vi "ADC SNR_original.vi"(8 "error in (no error)":errorcluster, 9 "Sequence parameters":string[][](array[string])=[["Min limit", "Max limit", "Register sheet file", "Register Sheet"], ["", "", "CC2600.xls", "TX_BLE;Trim"], ["Reg write (addr;value)", "Operating frequency [Hz]", "", ""], ["NA", "2.44G", "", ""]], 10 "Run type":i32, 11 "Method parameters":T4={"Dev"={"Do not disturb DUT"=FALSE, "XOSC"=32000000.0, "Board type"="", "EM"="", "Configure tempboard"=TRUE, "Device specific info"=[], "Generic Object"=refnum}, "Method"={"Run type"=1, "Test name"="Current LPM2 4", "Comment"="", "Results folder"="", "AFC"=enum."Off", "Method name"="Current LPM2 4", "Method results"={"Excel brief report"=FALSE, "Spotfire report"=FALSE, "Starfish report"=FALSE}, "Operator"="", "Reference time"=timestamp(0 s since 1904-01-01), "AFC delay"=0.0, "Initialization"=enum."Enabled", "MD5 Sum"="", "HW addon board"=enum."None", "AFC Regsheet"="", "AFC Regfile"=path "", "dummy"=0.0}, "Inst"={"Instr"={"PS1"={"Name"="", "GPIB address"="", "VISA session"=""}, "PS2"={"Name"="", "GPIB address"="", "VISA session"=""}, "TC1"={"Name"="", "GPIB address"="", "VISA session"=""}, "TC2"={"Name"="", "GPIB address"="", "VISA session"=""}, "SA1"={"Name"="", "GPIB address"="", "VISA session"=""}, "SA2"={"Name"="", "GPIB address"="", "VISA session"=""}, "SG1"={"Name"="", "GPIB address"="", "VISA session"=""}, "SG2"={"Name"="", "GPIB address"="", "VISA session"=""}, "SG3"={"Name"="", "GPIB address"="", "VISA session"=""}, "MI1"={"Name"="", "GPIB address"="", "VISA session"=""}, "MI2"={"Name"="", "GPIB address"="", "VISA session"=""}, "SW SA"={"Name"="", "Controller addr"=""}, "SW SG"={"Name"="", "Controller addr"=""}, "MI3"={"Name"="", "GPIB address"="", "VISA session"=""}}, "Switchbox"={"RF Path"=0, "Cal compensation"=enum."TX", "Switchbox gain mode"="", "State"=enum."TX"}, "Instr to control (i.e. SA1)"="Default", "Intrument info string"=""}, "Sequence parameters"=[["Weight", "Min Limit", "Max Limit", "Register Sheet", "", "", "", "", "", "", "", "", ""], ["Vital", "", "1", "LPM2", "", "", "", "", "", "", "", "", ""], ["Resolution", "Reg write (addr;value)", "Chip mode", "Range", "", "", "", "", "", "", "", "", ""], ["u", "NA", "", "auto", "", "", "", "", "", "", "", "", ""]], "Cond"={"Temp logged"=25.0, "VDD1_PS1_6V"=-999.0, "VDD2_PS1_25V"=-999.0, "VDD4_PS2_25V"=-999.0, "VDD3_PS2_6V"=-999.0}, "Meas config"={"X-axis inner loop index"=32000000, "Y-axis outer loop index"=32000000, "X-axis"=[], "Y-axis"=[], "X-axis array req size"=32000000, "Y-axis array req size"=32000000, "Param description"=[], "Use meas clust for reporting"=FALSE, "Parameter index (page)"=0, "X-axis name"="", "Y-axis name"=""}} {"Cond"."VDD3_PS2_6V" format="%.3f"; "Cond"."VDD4_PS2_25V" format="%.3f"; "Cond"."VDD2_PS1_25V" format="%.3f"; "Cond"."VDD1_PS1_6V" format="%.3f"; "Method"."dummy" format="%.1p"; "Method"."AFC delay" format="%.1p"; "Dev"."XOSC" format="%.3p"}) -> (0 "error out":errorcluster, 1 "End method error":T3, 3 "Result summary":string[][](array[string])=[["Critical", "Output Power@2405 MHz", "-3", "4", "dBm"], ["Critical", "Output Power@2410 MHz", "-3", "4", "dBm"]])   [LabVIEW 2019]
doc: "[AutoDocStart]Performs crystal accuracy measurements. Measures the offset from ideal frequency. Primarily used for tuning XOSC capacitors and verifying XOSC trims.\n\nSweeping parameters: operating frequency, OSC override value and VDDR level\n\nResults: Offset frequency in ppm[AutoDocEnd]"
uses:
  User Lib/Utilities/Cluster definitions/DUT VDD1.ctl
  User Lib/Utilities/Cluster definitions/DUT VDD2.ctl
  User Lib/Utilities/Cluster definitions/DUT VDD3.ctl
  User Lib/Utilities/Cluster definitions/DUT VDD4.ctl
  User Lib/Utilities/Cluster definitions/DUT vdd control.ctl
  User Lib/Utilities/Cluster definitions/Instr clust.ctl
  User Lib/Utilities/Cluster definitions/Method input.ctl
  User Lib/Utilities/Controls/Automatic Frequency Compensation types.ctl
  User Lib/Utilities/Controls/Method Reports.ctl
  User Lib/Utilities/Cluster definitions/End method error cluster.ctl
  User Lib/Utilities/Cluster definitions/Device specific info.ctl
  User Lib/Utilities/Cluster definitions/Method Initialization.ctl
  User Lib/Utilities/Switchbox control/SwitchBox_State._ENUMctl.ctl
  User Lib/Utilities/Controls/HW addon boards.ctl
panel:
  in  "path to save":T1={"Path to Save plot"=path "D:/Tenor_176P/DYN_PAR_C004/DAT/D001_TEMPP30C_VDD1.2_VDDA3.3_16B_SE_ADCA__vicA_aggX_PLT_CAP_200821_1740_33.jpg", "Path to Raw Data plot"=path "D:/Tenor_176P/DYN_PAR_C004/DAT/D001_TEMPP30C_VDD1.2_VDDA3.3_16B_SE_ADCA__vicA_aggX_RAW_DAT_200821_1740_33.csv"}
  in  "Tab Control":T2(tab)
  out "Dynamic Parameters":T12={"SNR"=nan, "SNRD"=nan, "THD"=nan, "ENOB (SNRD)"=nan, "SFDR"=nan, "ENOB (SNR)"=nan, "Noise Power"=nan, "Signal power"=nan} {"Signal power" format="%.6f"; "Noise Power" format="%.2f"; "ENOB (SNR)" format="%.2f"; "SFDR" format="%.2f"; "ENOB (SNRD)" format="%.2f"; "THD" format="%.2f"; "SNRD" format="%.2f"; "SNR" format="%.2f"}
  # "°C"
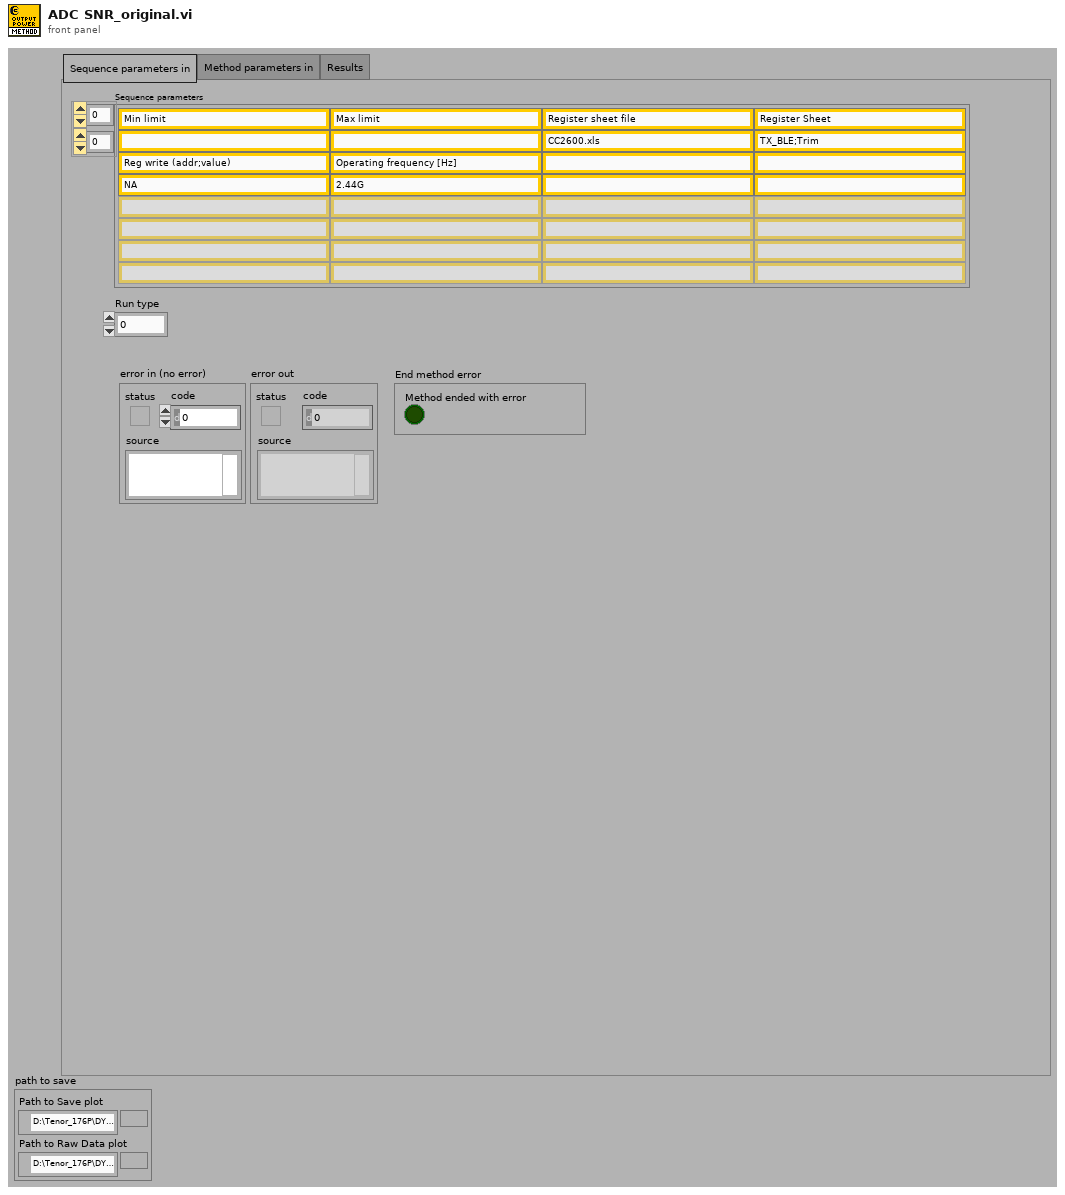
[diagram p1: front panel]
types:
  T1 = cluster{"Path to Save plot":path, "Path to Raw Data plot":path}
  T2 = enum32{"Sequence parameters in", "Method parameters in", "Results"}
  T3 = typedef "End method error cluster.ctl" = cluster{"Method ended with error":bool}
  T4 = typedef "Method input.ctl" = cluster{"Dev":cluster{"Do not disturb DUT":bool, "XOSC":dbl, "Board type":string, "EM":string, "Configure tempboard":bool, "Device specific info":T5[], "Generic Object":refnum<class>}, "Method":cluster{"Run type":i32, "Test name":string, "Comment":string, "Results folder":string, "AFC":T6, "Method name":string, "Method results":T7, "Operator":string, "Reference time":timestamp, "AFC delay":dbl, "Initialization":T8, "MD5 Sum":string, "HW addon board":T9, "AFC Regsheet":string, "AFC Regfile":path, "dummy":dbl}, "Inst":T10, "Sequence parameters":string[][], "Cond":cluster{"Temp logged":dbl, "VDD1_PS1_6V":dbl, "VDD2_PS1_25V":dbl, "VDD4_PS2_25V":dbl, "VDD3_PS2_6V":dbl}, "Meas config":cluster{"X-axis inner loop index":i32, "Y-axis outer loop index":i32, "X-axis":string[], "Y-axis":string[], "X-axis array req size":i32, "Y-axis array req size":i32, "Param description":string[][], "Use meas clust for reporting":bool, "Parameter index (page)":i32, "X-axis name":string, "Y-axis name":string}}
  T5 = typedef "Device specific info.ctl" = cluster{"EM number":u8, "IP address":string, "Enabled":bool, "Slot no":u8, "RF path":u8, "EM name":string, "Wafer info":string, "AFC frequency ppm":dbl, "Register writes":string[][], "Meas data":string[][][], "Device comment":string}
  T6 = typedef "Automatic Frequency Compensation types.ctl" = enum16{"Off", "Compensate Instrument frequency", "Compensate DUT frequency", "Predictive - Compensate Instrument frequency", "Predictive - Compensate DUT frequency", "Do not skip re-init - Compensate Instrument frequency", "Do not skip re-init - Compensate DUT frequency"}
  T7 = typedef "Method Reports.ctl" = cluster{"Excel brief report":bool, "Spotfire report":bool, "Starfish report":bool}
  T8 = typedef "Method Initialization.ctl" = enum16{"Enabled", "Skip Instr and Device Init", "Enabled with Separate Flash", "Set PS, Device Init and Skip Instr Init", "Skip Device Init"}
  T9 = typedef "HW addon boards.ctl" = enum16{"None", "Current meas 5EM", "Stresstest 10EM"}
  T10 = typedef "Instr clust.ctl" = cluster{"Instr":cluster{"PS1":cluster{"Name":string, "GPIB address":string, "VISA session":refnum<visa-resource-name>}, "PS2":cluster{"Name":string, "GPIB address":string, "VISA session":refnum<visa-resource-name>}, "TC1":cluster{"Name":string, "GPIB address":string, "VISA session":refnum<visa-resource-name>}, "TC2":cluster{"Name":string, "GPIB address":string, "VISA session":refnum<visa-resource-name>}, "SA1":cluster{"Name":string, "GPIB address":string, "VISA session":refnum<visa-resource-name>}, "SA2":cluster{"Name":string, "GPIB address":string, "VISA session":refnum<visa-resource-name>}, "SG1":cluster{"Name":string, "GPIB address":string, "VISA session":refnum<visa-resource-name>}, "SG2":cluster{"Name":string, "GPIB address":string, "VISA session":refnum<visa-resource-name>}, "SG3":cluster{"Name":string, "GPIB address":string, "VISA session":refnum<visa-resource-name>}, "MI1":cluster{"Name":string, "GPIB address":string, "VISA session":refnum<visa-resource-name>}, "MI2":cluster{"Name":string, "GPIB address":string, "VISA session":refnum<visa-resource-name>}, "SW SA":cluster{"Name":string, "Controller addr":string}, "SW SG":cluster{"Name":string, "Controller addr":string}, "MI3":cluster{"Name":string, "GPIB address":string, "VISA session":refnum<visa-resource-name>}}, "Switchbox":cluster{"RF Path":i32, "Cal compensation":enum16{"TX", "RX", "Interferer", "No compensation", "Interferer2"}, "Switchbox gain mode":string, "State":T11}, "Instr to control (i.e. SA1)":string, "Intrument info string":string}
  T11 = typedef "SwitchBox_State._ENUMctl.ctl" = enum16{"TX", "RX", "SP:TX", "SP:RX", "SW:TX", "SW:RX"}
  T12 = cluster{"SNR":dbl, "SNRD":dbl, "THD":dbl, "ENOB (SNRD)":dbl, "SFDR":dbl, "ENOB (SNR)":dbl, "Noise Power":dbl, "Signal power":dbl}
  T13 = cluster{"Save INL/DNL Plot(Ramp)":bool, "Save SNR Plot":bool, "Save INL/DNL Plot(Sine)":bool, "Save INL/DNL Raw Data(Ramp)":bool, "Save SNR Raw Data":bool, "Save INL/DNL Raw Data(Sine)":bool, "Save DC Raw data":bool, "Save  Raw Data(Sine)":bool}
  T14 = cluster{"Fundamental Frequency":dbl, "Sampling Frequncy":dbl, "No of Harmonics":u8, "Window":enum16{"None ", "Hanning", "Hamming", "Blackman-Harris", "Exact Blackman", "Blackman", "Flat Top", "4 Term B-Harris ", "7 Term B-Harris"}, "Blackman (fundamental power) bins)":dbl}
  T15 = typedef "DUT vdd control.ctl" = cluster{"VDD4 config":T16, "VDD3 config":T17, "VDD2 config":T18, "VDD1 config":T19}
  T16 = typedef "DUT VDD4.ctl" = u16
  T17 = typedef "DUT VDD3.ctl" = u16
  T18 = typedef "DUT VDD2.ctl" = u16
  T19 = typedef "DUT VDD1.ctl" = u16
  T20 = enum32{"NI Card Settings", "Memory Read Setting", "DC Capture", "ADC Ramp", "ADC Sine", "SNR", "Cap Calibration"}
  T21 = enum32{"Read from Memory", "Read .dat file", "NI Card Capture", "None"}
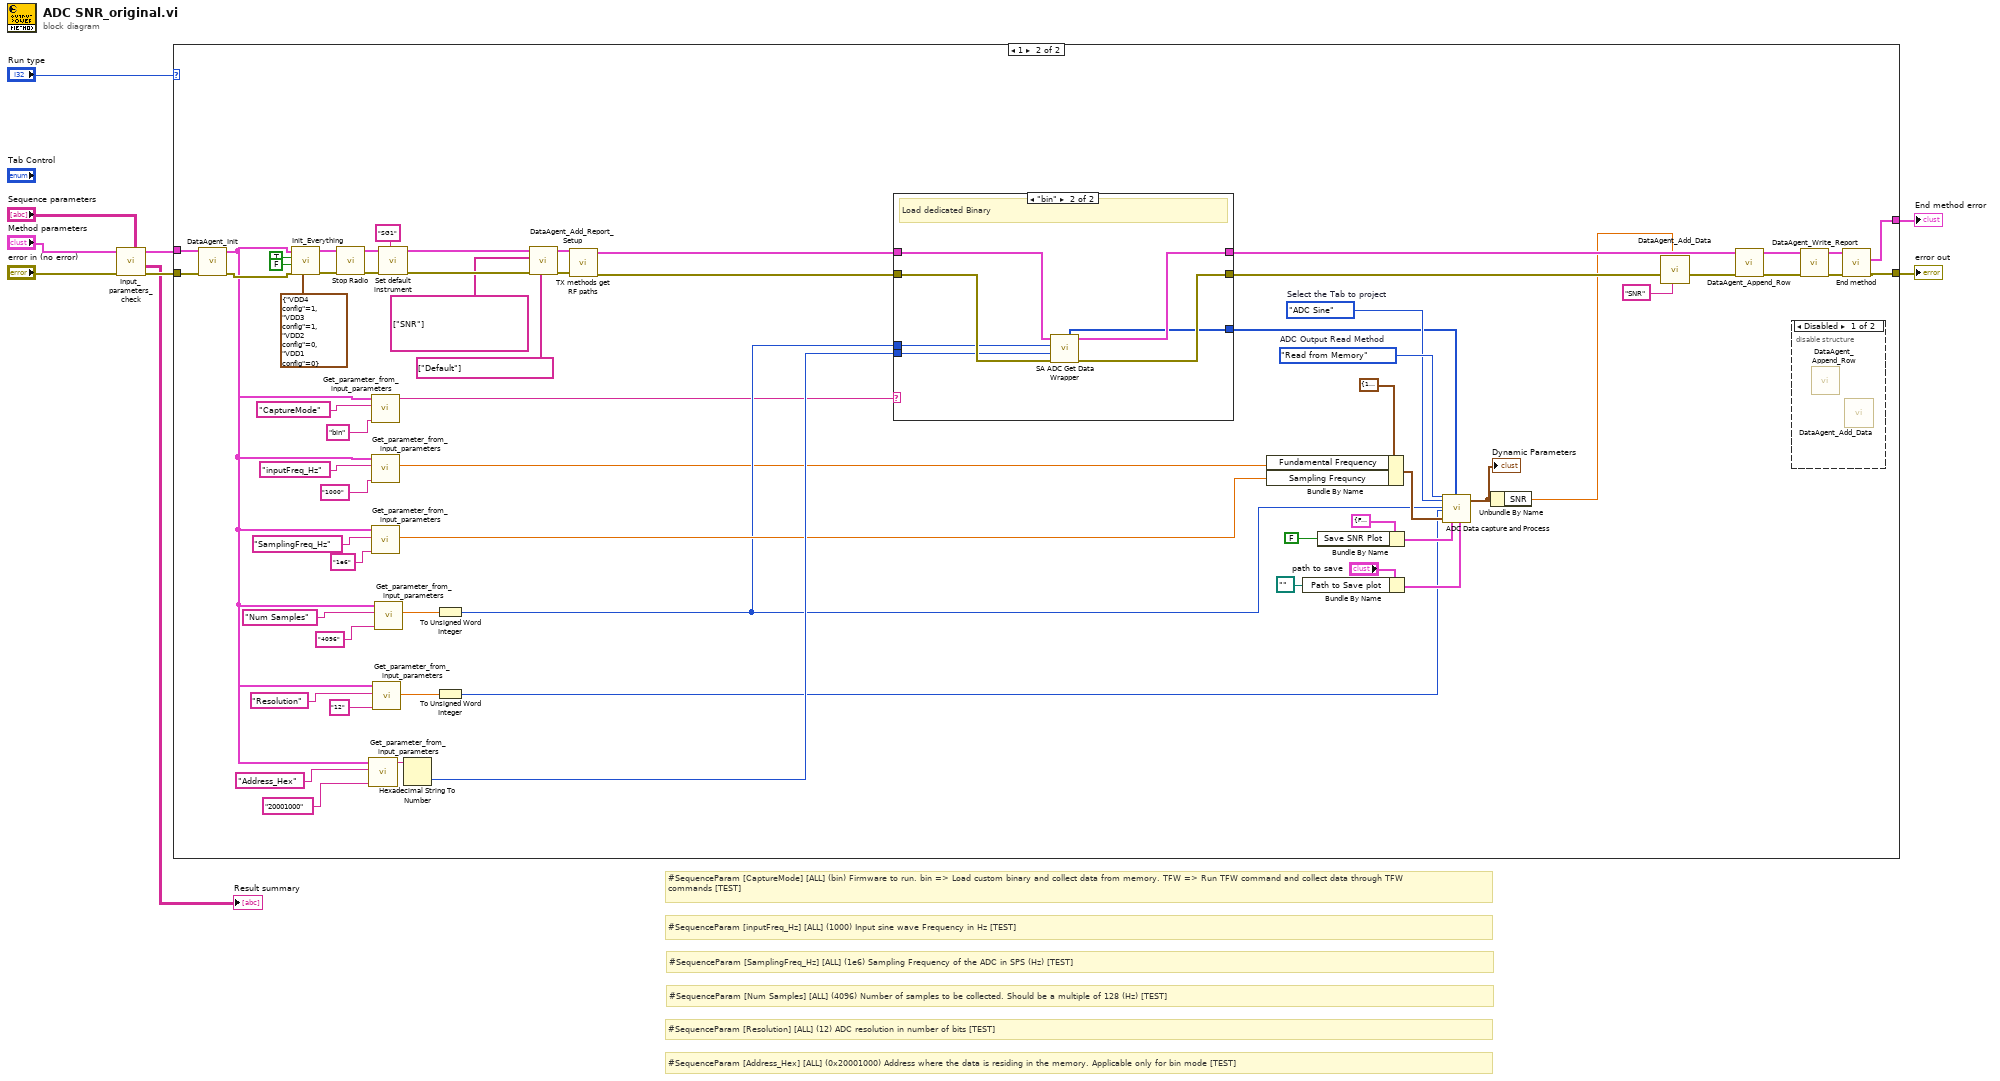
[diagram p0: block diagram]
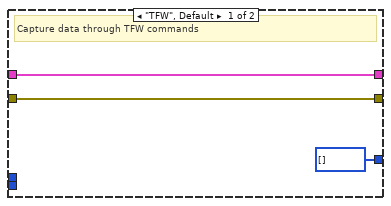
[diagram p3: hidden frame]
diagram:
  # "#SequenceParam [CaptureMode] [ALL] (bin) Firmware to run. bin => Load custom binary and collect data from memory. TFW => Run TFW command and collect data through TFW commands [TEST]"
  # "#SequenceParam [Address_Hex] [ALL] (0x20001000) Address where the data is residing in the memory. Applicable only for bin mode [TEST]"
  # "#SequenceParam [Resolution] [ALL] (12) ADC resolution in number of bits [TEST]"
  # "#SequenceParam [Num Samples] [ALL] (4096) Number of samples to be collected. Should be a multiple of 128 (Hz) [TEST]"
  # "#SequenceParam [SamplingFreq_Hz] [ALL] (1e6) Sampling Frequency of the ADC in SPS (Hz) [TEST]"
  # "#SequenceParam [inputFreq_Hz] [ALL] (1000) Input sine wave Frequency in Hz [TEST]"
  n1 = call "Input_parameters_check.vi"("Sequence parameters"="Sequence parameters", "error in"="error in (no error)", "Method cluster in"="Method parameters") -> ("error out"=w8:errorcluster, "Result summary"=→"Result summary":string[][], "Method cluster out"=w4:T4)  [unwired: 6 in]
  n2 = case shown="1" "Run type" {
    tunnel: w8 -> [w10 w67]
    tunnel: [w10 w74] -> w9
    tunnel: w4 -> [_ w68]
    tunnel: [_ w73] -> w3
    frame 0, Default {
      # "Run type 0 is only for formatting the result summary"
    }
    frame 1 {
      w37 = T20."ADC Sine"  # Select the Tab to project
      w38 = T21."Read from Memory"  # ADC Output Read Method
      n3 = call "DataAgent_Init.vi"("error in (no error)"=w67, "Method cluster in"=w68) -> ("error out"=w66:errorcluster, "Method cluster out"=w20:T4)  [unwired: 8 in]
      n4 = call "Init_Everything.vi"("VDD config"=T15 {"VDD4 config"=1, "VDD3 config"=1, "VDD2 config"=0, "VDD1 config"=0}, "error in"=w66, "Support current measurement?"=FALSE, "Override VDD Config"=TRUE, "Method cluster In"=w20) -> ("error out"=w59:errorcluster, "Method cluster out"=w56:T4)  [unwired: 3 in, 2 out]
      n5 = call "Stop Radio.vi"("error in (no error)"=w59, "Method cluster in"=w56) -> ("error out"=w58:errorcluster, "Method cluster out"=w57:T4)  [unwired: 8 in]
      n6 = call "Get_parameter_from_input_parameters.vi"("Default value (used if not specified on Front Panel)"="20001000", "Parameter name"="Address_Hex" ("SA_ param name"), "Method cluster (if input param empty)"=w20) -> ("value as String"=w43:string)  [unwired: 2 in, 6 out]
      n7 = call "Get_parameter_from_input_parameters.vi"("Default value (used if not specified on Front Panel)"="bin", "Parameter name"="CaptureMode" ("SA_ param name"), "Method cluster (if input param empty)"=w20) -> ("value as String"=w19:string)  [unwired: 2 in, 6 out]
      n8 = call "Get_parameter_from_input_parameters.vi"("Default value (used if not specified on Front Panel)"="1000", "Parameter name"="inputFreq_Hz" ("SA_ param name"), "Method cluster (if input param empty)"=w20) -> ("value as DBL"=w23:dbl)  [unwired: 2 in, 6 out]
      n9 = call "Get_parameter_from_input_parameters.vi"("Default value (used if not specified on Front Panel)"="1e6", "Parameter name"="SamplingFreq_Hz" ("SA_ param name"), "Method cluster (if input param empty)"=w20) -> ("value as DBL"=w39:dbl)  [unwired: 2 in, 6 out]
      n10 = call "Get_parameter_from_input_parameters.vi"("Default value (used if not specified on Front Panel)"="12", "Parameter name"="Resolution" ("SA_ param name"), "Method cluster (if input param empty)"=w20) -> ("value as DBL"=w45:dbl)  [unwired: 2 in, 6 out]
      n11 = call "Get_parameter_from_input_parameters.vi"("Default value (used if not specified on Front Panel)"="4096", "Parameter name"="Num Samples" ("SA_ param name"), "Method cluster (if input param empty)"=w20) -> ("value as DBL"=w44:dbl)  [unwired: 2 in, 6 out]
      n12 = call "Set default instrument.vi"("Default value (used if not specified on Front Panel)"="SG1", "error in (no error)"=w58, "Method cluster in"=w57) -> ("error out"=w65:errorcluster, "Method cluster out"=w64:T4)  [unwired: 7 in]
      n13 = Hexadecimal String To Number(string=w43) -> (number=w42:u32)  [unwired: 2 in, 1 out]
      n14 = To Unsigned Word Integer(number=w44) -> (unsigned 16bit integer=w27:u16)
      n15 = To Unsigned Word Integer(number=w45) -> (unsigned 16bit integer=w26:u16)
      n16 = call "DataAgent_Add_Report_Setup.vi"("Y-axis Titles"=string[] ["Default"], "error in (no error)"=w65, "Loop parameter names"=string[] ["SNR"], "Method cluster in"=w64) -> ("error out"=w52:errorcluster, "Method cluster out"=w53:T4)  [unwired: 3 in, 3 out]
      n17 = call "TX methods get RF paths.vi"("error in (no error)"=w52, "Method clust in"=w53) -> ("error out"=w55:errorcluster, "Method clust out"=w54:T4)  [unwired: 7 in, 1 out]
      n18 = case shown="\"bin\"" w19 {
        tunnel: [w77 w84] -> w18
        tunnel: [w76 w83] -> w15
        tunnel: w55 -> [w76 w82]
        tunnel: w54 -> [w77 w81]
        tunnel: w42 -> [_ w80]
        tunnel: [u32[] [] ("ADC samples") w79] -> w31
        tunnel: w27 -> [_ w78]
        frame "TFW", Default {
          # "Capture data through TFW commands"
        }
        frame "bin" {
          # "Load dedicated Binary"
          n19 = call "SA ADC Get Data Wrapper.vi"("error in"=w82, "Data Address"=w80, "Num Samples"=w78, "Method cluster in"=w81) -> ("error out"=w83:errorcluster, "output cluster"=w84:T4, "ADC samples"=w79:u32[])  [unwired: 2 in, 3 out]
        }
      }
      n20 = Bundle By Name(cluster=T14 {"Fundamental Frequency"=100000.0, "Sampling Frequncy"=3999610.0, "No of Harmonics"=9, "Window"=enum."7 Term B-Harris", "Blackman (fundamental power) bins)"=1.0} ("Inputs for Dyanmic para"), "Fundamental Frequency"=w23, "Sampling Frequncy"=w39) -> (w34:T14)
      n21 = Bundle By Name(cluster="path to save", "Path to Save plot"=path "") -> (w29:T1)
      n22 = Bundle By Name(cluster=T13 {"Save INL/DNL Plot(Ramp)"=FALSE, "Save SNR Plot"=FALSE, "Save INL/DNL Plot(Sine)"=FALSE, "Save INL/DNL Raw Data(Ramp)"=FALSE, "Save SNR Raw Data"=FALSE, "Save INL/DNL Raw Data(Sine)"=FALSE, "Save DC Raw data"=FALSE, "Save  Raw Data(Sine)"=FALSE} ("Save data"), "Save SNR Plot"=FALSE) -> (w33:T13)
      n23 = call "ADC Data capture and Process.vi"("ADC Output Read Method"=w38, "Select the Tab to project"=w37, "No.of samples"=w27, "Resolution"=w26, "Inputs for Dyanmic para"=w34, "Save data"=w33, "Input Waveform"=w31, "path to save"=w29) -> ("Dynamic Parameters"=w12:T12)  [unwired: 14 in, 5 out]
      "Dynamic Parameters" <- w12
      n24 = Unbundle By Name(w12) -> ("SNR"=w11:dbl)
      n25 = call "DataAgent_Add_Data.vi"("ColumnName"="SNR" ("Default Value"), "Data"=w11, "error in (no error)"=w15) -> ("error out"=w14:errorcluster)  [unwired: 8 in]
      n26 = call "DataAgent_Append_Row.vi"("error in (no error)"=w14, "Method cluster in"=w18) -> ("error out"=w16:errorcluster, "Method cluster out"=w17:T4)  [unwired: 8 in]
      n27 = disable-structure shown="Disabled" {
        frame Disabled {
          n28 = call "DataAgent_Append_Row.vi"() -> ()  [unwired: 10 in, 2 out]
          n29 = call "DataAgent_Add_Data.vi"() -> ()  [unwired: 11 in, 1 out]
        }
        frame Enabled {
        }
      }
      n30 = call "DataAgent_Write_Report.vi"("error in (no error)"=w16, "Method cluster in"=w17) -> ("error out"=w63:errorcluster, "Method cluster out"=w62:T4)  [unwired: 8 in]
      n31 = call "End method.vi"("error in"=w63, "Method cluster in"=w62) -> ("error out"=w74:errorcluster, "End method error"=w73:T3)  [unwired: 7 in, 1 out]
    }
  }
  "error out" <- w9
  "End method error" <- w3
